vi "Read TemporalData.vi"(8 "error in (no error)":errorcluster, 10 "ReadSize":u32, 11 "AODAcq in":refnum<class "AODAcq.lvclass">) -> (0 "error out":errorcluster, 2 "TemporalData":waveform(i32)[](array[waveform]), 3 "AODAcq out":refnum<class "AODAcq.lvclass">)   [LabVIEW 2011, in "AODAcq.lvclass"]
uses:
  AODAcq.lvclass
  AODAcq.lvclass/AODAcq.ctl
  <instrlib>/niHWS/nihws.llb/niHWS Set Wfm DBL Attribute ID.ctl
  <vilib>/Utility/error.llb/Error Cluster From Error Code.vi
  <vilib>/rvi/errors/niLvFpgaAdjustHostInterfaceError.vi
  <instrlib>/niHWS/nihws.llb/niHWS Write Analog I32.vi
  <vilib>/rvi/interface/nirviMethod/nirviMethod.xnode
  FPGA_Control/AODRef.ctl
  FPGA_Control/FPGA Bitfiles/AODControl_FPGATarget_5751Acquire_F1CF9257.lvbitx
  FPGA_Control/AOD Control (FPGA).vi
  <vilib>/FPGAPlugInAG/PXIe-7965R/niLvFpga_ReadFifo_PXIe-7965R.vi
  <vilib>/rvi/errors/niLvFpgaMergeErrorWithErrorCode.vi
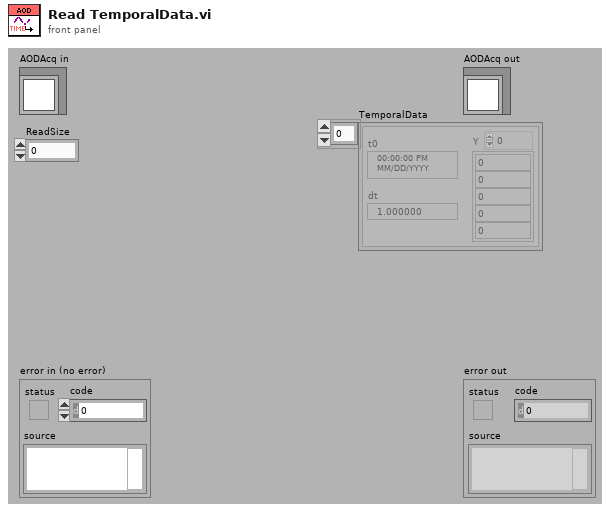
[diagram p1: front panel]
types:
  T1 = typedef "AODRef.ctl" = refnum<k20>
  T2 = typedef "niHWS Set Wfm DBL Attribute ID.ctl" = u32
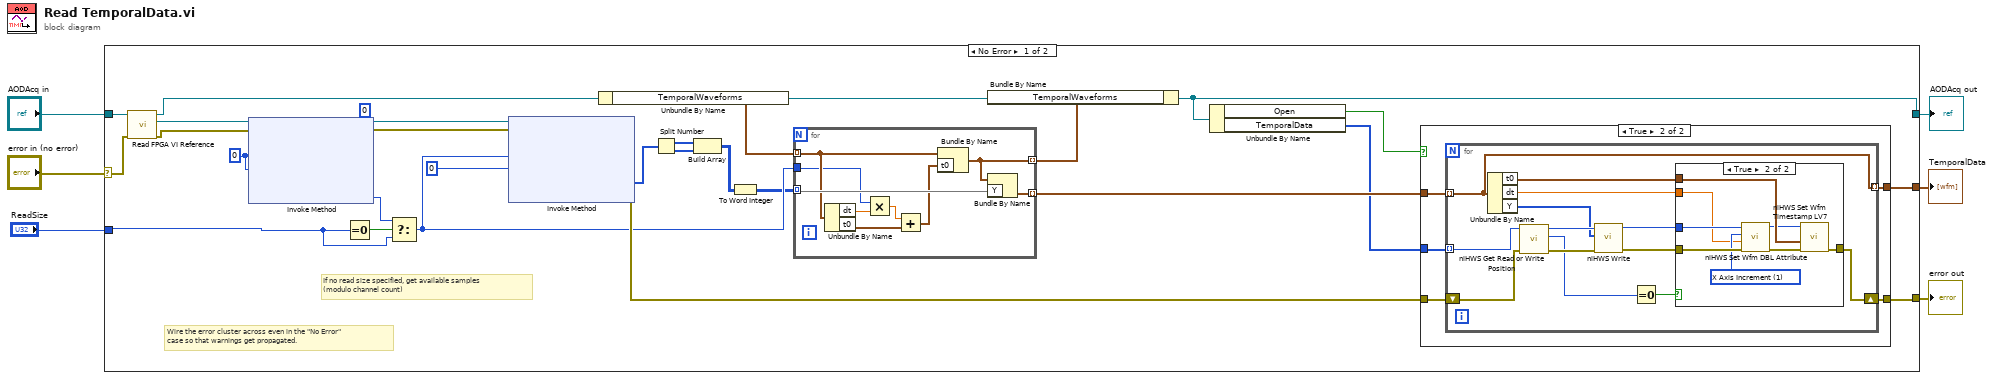
[diagram p0: block diagram]
diagram:
  n1 = case shown="No Error" "error in (no error)" {
    selector: "error in (no error)" -> [w27 w73]
    tunnel: [w18 w73] -> w5
    tunnel: [w22 w72] -> w3
    tunnel: "AODAcq in" -> [w33 w72]
    tunnel: "ReadSize" -> [w16 _]
    tunnel: [w17 _] -> w1
    frame No Error {
      (unwired) u32 0 ("y")
      w32 = u32 0 ("Number of Elements")
      # "If no read size specified, get available samples \n(modulo channel count)"
      # "Wire the error cluster across even in the \"No Error\"\ncase so that warnings get propagated."
      n2 = call-dynamic "Read FPGA VI Reference.vi"("error in (no error)"=w27, "AODAcq in"=w33) -> ("error out"=w8:errorcluster, "FPGA VI Reference"=w9:T1, "AODAcq out"=w25:refnum<class "AODAcq.lvclass">)  [unwired: 7 in]
      n3 = xnode "Invoke Method"("FPGA VI Reference In"=w9, "error in"=w8, "Number of Elements"=w32, "Timeout (ms)"=w32) -> ("FPGA VI Reference Out"=w30:T1, "error out"=w29:errorcluster, "Elements Remaining"=w15:u32)  [unwired: 1 out]
      n4 = Equal To 0?(x=w16) -> (x = 0?=w31:bool)
      n5 = Select(t=w15, s=w31, f=w16) -> (s? t:f=w10:u32)
      n6 = xnode "Invoke Method"("FPGA VI Reference In"=w30, "error in"=w29, "Number of Elements"=w10, "Timeout (ms)"=0) -> ("error out"=w19:errorcluster, "Data"=w14:i32[])  [unwired: 2 out]
      n7 = Unbundle By Name(w25) -> ("TemporalWaveforms"=w26:waveform(i32)[])
      n8 = Split Number(x=w14) -> (hi(x)=w12:u16[], lo(x)=w13:u16[])
      n9 = Build Array(w12, w13) -> (w11:u16[][])
      n10 = To Word Integer(number=w11) -> (16bit integer=w7:i16[][])
      n11 = for {
        tunnel: w7 -> [w71] mode=indexing
        tunnel: [w70] -> w23 mode=indexing
        tunnel: w26 -> [w66] mode=indexing
        tunnel: w10 -> [w63]
        tunnel: [w64] -> w24 mode=indexing
        n12 = Unbundle By Name(w66) -> ("dt"=w69:dbl, "t0"=w67:timestamp)
        n13 = Multiply(x=w63, y=w69) -> (x*y=w68:dbl)
        n14 = Add(x=w68, y=w67) -> (x+y=w65:timestamp)
        n15 = Bundle By Name(cluster=w66, "t0"=w65) -> (w64:waveform(i32))
        n16 = Bundle By Name(cluster=w64, "Y"=w71) -> (w70:waveform(i32))
      }
      n17 = Bundle By Name(cluster=w25, "TemporalWaveforms"=w24) -> (w22:refnum<class "AODAcq.lvclass">)
      n18 = Unbundle By Name(w22) -> ("Open"=w21:bool, "TemporalData"=w20:u32[])
      n19 = case shown="True" w21 {
        tunnel: w23 -> [w34 w40]
        tunnel: w20 -> [_ w39]
        tunnel: w19 -> [w35 w38]
        tunnel: [w35 w37] -> w18
        tunnel: [w34 w36] -> w17
        frame False {
        }
        frame True {
          n20 = for {
            tunnel: w40 -> [w41] mode=indexing
            tunnel: w39 -> [w45] mode=indexing
            shift-right: [w42] -> w37
            shift-left: w38 -> [w47]
            tunnel: [w41] -> w36 mode=indexing
            n21 = Unbundle By Name(w41) -> ("t0"=w43:timestamp, "dt"=w44:dbl, "Y"=w46:i32[])
            n22 = call <instrlib>:"niHWS Get Read or Write Position.vi"("waveform reference in"=w45, "error in (no error)"=w47) -> ("waveform reference out"=w52:u32, "position"=w49:u32, "error out"=w51:errorcluster)  [unwired: 6 out]
            n23 = call-poly <instrlib>:"niHWS Write.vi"("error in (no error)"=w51, "data"=w46, "waveform reference in"=w52) -> ("error out"=w50:errorcluster, "waveform reference out"=w53:u32)  [unwired: 7 in]
            n24 = Equal To 0?(x=w49) -> (x = 0?=w48:bool)
            n25 = case shown="True" w48 {
              tunnel: w43 -> [_ w61]
              tunnel: [w54 w60] -> w42
              tunnel: w50 -> [w54 w58]
              tunnel: w53 -> [_ w57]
              tunnel: w44 -> [_ w55]
              frame False {
              }
              frame True {
                w56 = T2 1 items=["X Axis Start"=0, "X Axis Increment"=1, "Y Axis Minimum"=3, "Y Axis Maximum"=4] ("Attribute ID")
                n26 = call <instrlib>:"niHWS Set Wfm DBL Attribute.vi"("error in (no error)"=w58, "attribute value"=w55, "attribute ID"=w56, "waveform reference in"=w57) -> ("error out"=w62:errorcluster, "waveform reference out"=w59:u32)  [unwired: 6 out]
                n27 = call <instrlib>:"niHWS Set Wfm Timestamp LV7.vi"("error in (no error)"=w62, "waveform timestamp"=w61, "waveform reference in"=w59) -> ("error out"=w60:errorcluster)  [unwired: 8 out]
              }
            }
          }
        }
      }
    }
    frame Error {
    }
  }
  "error out" <- w5
  "AODAcq out" <- w3
  "TemporalData" <- w1
